vi "RT Loop - System Health and FPGA Monitoring.vi"(11 "Message Queue":refnum<queue>) -> ()   [LabVIEW 2014]
uses:
  support/Message Queue/Message Cluster.ctl
  controls/FPGA VI Reference.ctl
  Globals/Global - Configuration Options.vi
  Globals/Global - All RT Loop Stop.vi
  Globals/Global - Monitoring Variables.vi
  <vilib>/Utility/error.llb/Error Cluster From Error Code.vi
  <vilib>/rvi/errors/niLvFpgaAdjustHostInterfaceError.vi
  <vilib>/nisyscfg/Close (System).vi
  <vilib>/rvi/interface/nirviReadWriteControl/nirviReadWriteControl.xnode
  <vilib>/NI_Real-Time Target Support.lvlib
  <vilib>/nisyscfg/nisyscfg.lvlib
  <resource>/objmgr/nisysapi.rc
  NiFpgaLv.dll
  <vilib>/rvi/interface/Simulation/niFpgaSimulationCallBeginRW.vi
  support/Message Queue/Message Queue.lvlib
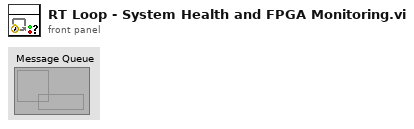
[diagram p1: front panel]
types:
  T1 = typedef "FPGA VI Reference.ctl" = refnum<k20>
  T2 = typedef "NI_Real-Time Target Support.lvlib/RT CPU Load.ctl" = cluster{"Total (%)":dbl, "Time Critical (%)":dbl, "Timed Structures (%)":dbl, "High (%)":dbl, "Above Normal (%)":dbl, "Normal (%)":dbl, "Background (%)":dbl, "Idle (%)":dbl, "ISR (%)":dbl}
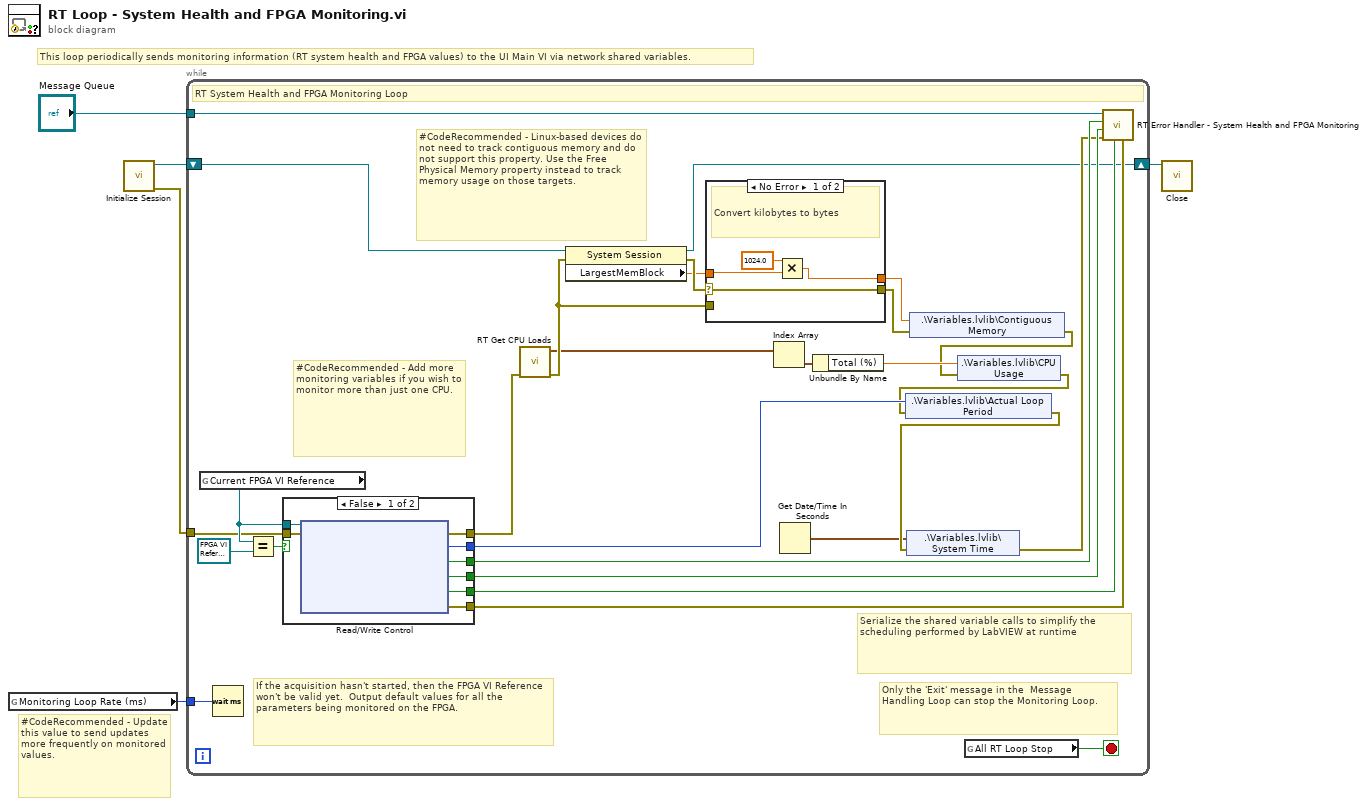
[diagram p0: block diagram]
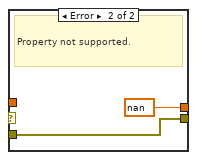
[diagram p2: hidden frame]
diagram:
  # "#CodeRecommended - Update this value to send updates more frequently on monitored values."
  # "This loop periodically sends monitoring information (RT system health and FPGA values) to the UI Main VI via network shared variables."
  n1 = global read "Global - Configuration Options.vi" "Monitoring Loop Rate (ms)"() -> (w4:u32)
  n2 = call <vilib>:"Initialize Session.vi"() -> ("error out"=w1:errorcluster, "Session out"=w3:refnum<k21>)  [unwired: 10 in]
  n3 = while {
    tunnel: "Message Queue" -> [w28]
    tunnel: w4 -> [w27]
    shift-right: [w12] -> w2
    shift-left: w3 -> [w13]
    tunnel: w1 -> [w9]
    stop <- w29 stop-if-true
    # "#CodeRecommended - Linux-based devices do not need to track contiguous memory and do not support this property. Use the Free Physical Memory property instead to track memory usage on those targets."
    # "#CodeRecommended - Add more monitoring variables if you wish to monitor more than just one CPU."
    # "If the acquisition hasn't started, then the FPGA VI Reference won't be valid yet.  Output default values for all the parameters being monitored on the FPGA."
    # "Serialize the shared variable calls to simplify the scheduling performed by LabVIEW at runtime"
    # "Only the 'Exit' message in the  Message Handling Loop can stop the Monitoring Loop."
    # "RT System Health and FPGA Monitoring Loop"
    n4 = global read "Global - Monitoring Variables.vi" "Current FPGA VI Reference"() -> (w19:T1)
    n5 = Wait (ms)(milliseconds to wait=w27) -> ()  [unwired: 1 out]
    n6 = Equal?(x=w19, y=T1 refnum ("Current FPGA VI Reference")) -> (x = y?=w17:bool)
    n7 = case shown="False" w17 {
      tunnel: [w47 _] -> w26
      tunnel: [w40 _] -> w25
      tunnel: [w46 _] -> w24
      tunnel: [w45 _] -> w23
      tunnel: [w44 _] -> w22
      tunnel: [w43 _] -> w21
      tunnel: w19 -> [w42 _]
      tunnel: w9 -> [w41 _]
      frame False {
        n8 = xnode "Read/Write Control"("FPGA VI Reference In"=w42, "error in"=w41) -> ("error out"=w47:errorcluster, "Sample Period (uSec)"=w40:u32, "Sample Gated"=w46:bool, "DMA FIFO Full"=w45:bool, "Different Channel Count"=w44:bool, "FPGA Error"=w43:errorcluster)  [unwired: 1 out]
      }
      frame True {
      }
    }
    n9 = call <vilib>:"RT Get CPU Loads.vi"("error in (no error)"=w26) -> ("error out"=w33:errorcluster, "CPU loads"=w31:T2[])  [unwired: 9 in]
    n10 = property class="System Session"(reference=w13, error in=w33) -> (reference out=w12:refnum<k21>, error out=w32:errorcluster, "LargestMemBlock"=w6:dbl)
    n11 = case shown="No Error" w32 {
      selector: w32 -> [w34 _]
      tunnel: w6 -> [w36 _]
      tunnel: [w35 nan] -> w8
      tunnel: [w34 w38] -> w7
      tunnel: w33 -> [_ w38]
      frame No Error {
        # "Convert kilobytes to bytes"
        n12 = Multiply(x=1024.0, y=w36) -> (x*y=w35:dbl)
      }
      frame Error {
        # "Property not supported."
      }
    }
    n13 = Index Array(array=w31) -> (element=w30:T2)  [unwired: 1 in]
    n14 = Get Date/Time In Seconds() -> (seconds since 1Jan1904=w14:timestamp)
    n15 = Unbundle By Name(w30) -> ("Total (%)"=w16:dbl)
    n16 = shared-variable ".\\Variables.lvlib\\Contiguous Memory"(w8, error in=w7) -> (error out=w11:errorcluster)
    n17 = shared-variable ".\\Variables.lvlib\\CPU Usage"(w16, error in=w11) -> (error out=w10:errorcluster)
    n18 = shared-variable ".\\Variables.lvlib\\Actual Loop Period"(w25, error in=w10) -> (error out=w20:errorcluster)
    n19 = shared-variable ".\\Variables.lvlib\\System Time"(w14, error in=w20) -> (error out=w15:errorcluster)
    n20 = global read "Global - All RT Loop Stop.vi" "All RT Loop Stop"() -> (w29:bool)
    n21 = call "RT Error Handler - System Health and FPGA Monitoring.vi"("FPGA Error (FPGA)"=w21, "Different Channel Count (FPGA)"=w22, "error in (no error)"=w15, "DMA FIFO Full (FPGA)"=w23, "Sample Gated (FPGA)"=w24, "Message Queue"=w28) -> ()  [unwired: 5 in, 1 out]
  }
  n22 = call-poly <vilib>:"Close.vi"("Session in"=w2) -> ()  [unwired: 10 in, 1 out]
